vi "Current Motors with Encoder State.vi"(8 "error in (no error)":errorcluster, 10 "Motors with Encoder State":T1={"Forward Switch"=FALSE, "Reverse Switch"=FALSE, "Measured RPM"=0.0, "Distance (in)"=0.0, "Setpoint RPM"=0.0, "Encoder Count"=0, "Home Count"=0, "Config"={"Counts  Per Revolution"=0, "Invert Encoder Direction"=FALSE, "Diameter of Revolution"=0.0, "Max RPM"=0.0, "Encoder Control"=TRUE}}, 11 "Elevator in":refnum<class "Elevator.lvclass">) -> (0 "error out":errorcluster, 3 "Elevator out":refnum<class "Elevator.lvclass">)   [LabVIEW 2014, in "Elevator.lvlib" / "Elevator.lvclass"]
uses:
  Elevator.lvclass
  Motor with Encoders/Motors with Encoders Class/Motors with Encoders State.ctl
  Motor with Encoders/Motors with Encoders Class/Motors with Encoders Config.ctl
  Elevator.lvclass/Elevator.ctl
  <vilib>/ActorFramework/Message Enqueuer/Message Enqueuer.lvclass/Message Enqueuer.ctl
  <vilib>/ActorFramework/Message Enqueuer/Enqueue.vi
  <vilib>/ActorFramework/Message Priority Queue/Priority Enqueue.vi
  Motor with Encoders/Motors with Encoders Messages/Zero Distance Msg/Zero Distance Msg.lvclass
  Motor with Encoders/Motors with Encoders Class/Motors with Encoders.lvclass
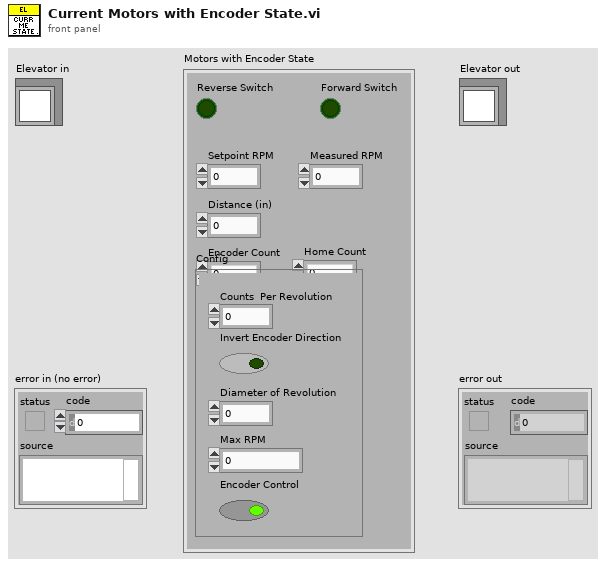
[diagram p1: front panel]
types:
  T1 = typedef "Motors with Encoders.lvlib/Motors with Encoders.lvclass/Motors with Encoders State.ctl" = cluster{"Forward Switch":bool, "Reverse Switch":bool, "Measured RPM":dbl, "Distance (in)":dbl, "Setpoint RPM":dbl, "Encoder Count":i64, "Home Count":i64, "Config":T2}
  T2 = typedef "Motors with Encoders.lvlib/Motors with Encoders.lvclass/Motors with Encoders Config.ctl" = cluster{"Counts  Per Revolution":u32, "Invert Encoder Direction":bool, "Diameter of Revolution":dbl, "Max RPM":dbl, "Encoder Control":bool}
  T3 = typedef "Elevator.lvlib/Elevator.lvclass/Elevator State.ctl" = cluster{"At Bottom":bool, "At Top":bool, "At Setpoint":bool, "Target Rate (RPM)":dbl, "Current Travel Rate":dbl, "Current Elevation":dbl, "Brake On":bool, "Motor Elevate Rate (RPM))":dbl, "Has Been Home":bool}
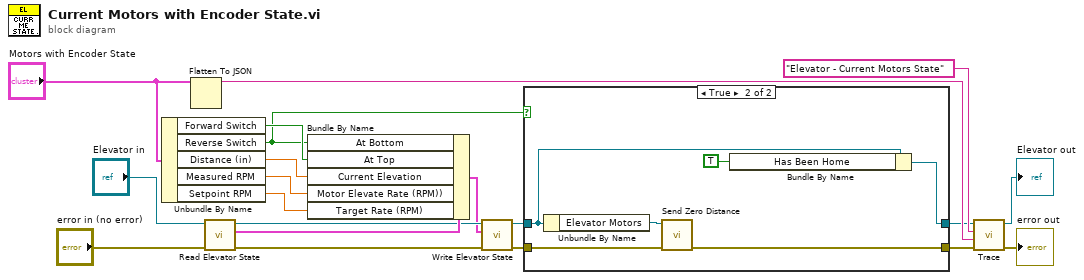
[diagram p0: block diagram]
diagram:
  n1 = Unbundle By Name("Motors with Encoder State") -> ("Forward Switch"=w15:bool, "Reverse Switch"=w4:bool, "Distance (in)"=w13:dbl, "Measured RPM"=w8:dbl, "Setpoint RPM"=w1:dbl)
  n2 = Flatten To JSON(anything="Motors with Encoder State") -> (JSON string=w9:string)  [unwired: 2 in, 1 out]
  n3 = call-dynamic "Read Elevator State.vi"("error in (no error)"="error in (no error)", "Elevator in"="Elevator in") -> ("error out"=w20:errorcluster, "Elevator State"=w19:T3, "Elevator out"=w18:refnum<class "Elevator.lvclass">)  [unwired: 7 in]
  n4 = Bundle By Name(cluster=w19, "At Bottom"=w4, "At Top"=w15, "Current Elevation"=w13, "Motor Elevate Rate (RPM))"=w8, "Target Rate (RPM)"=w1) -> (w16:T3)
  n5 = call-dynamic "Write Elevator State.vi"("error in (no error)"=w20, "Elevator State"=w16, "Elevator in"=w18) -> ("error out"=w7:errorcluster, "Elevator out"=w5:refnum<class "Elevator.lvclass">)  [unwired: 7 in]
  n6 = case shown="True" w4 {
    tunnel: w7 -> [w22 w27]
    tunnel: [w22 w26] -> w6
    tunnel: w5 -> [w21 w25]
    tunnel: [w21 w24] -> w3
    frame False {
    }
    frame True {
      n7 = Unbundle By Name(w25) -> ("Elevator Motors"=w28:refnum<class "Message Enqueuer.lvclass">)
      n8 = call "Send Zero Distance.vi"("error in (no error)"=w27, "Message Enqueuer"=w28) -> ("error out"=w26:errorcluster)  [unwired: 8 in, 1 out]
      n9 = Bundle By Name(cluster=w25, "Has Been Home"=TRUE ("Elevator State.Has Been Home")) -> (w24:refnum<class "Elevator.lvclass">)
    }
  }
  n10 = call-dynamic "Trace.vi"("error in (no error)"=w6, "System Message"=w9, "System Action"="Elevator - Current Motors State", "System Actor in"=w3) -> ("error out"=→"error out":errorcluster, "System Actor out"=→"Elevator out":refnum<class "Elevator.lvclass">)  [unwired: 6 in]
